vi "9239_1.vi"() -> ()   [LabVIEW 2014]
uses:
  <vilib>/Platform/TimedLoop/XDataNode/timing_clust.ctl
  <vilib>/Platform/TimedLoop/XDataNode/nitl_modes.ctl
  <vilib>/Platform/TimedLoop/XDataNode/wakeup.ctl
  <vilib>/Platform/TimedLoop/XDataNode/XDataNode.xnode
  <vilib>/Platform/TimedLoop/XDataNode/XDNodeRunTimeDep.lvlib
panel:
  out "已采样数量":dbl
  out "a1通道零漂采集":dynamicdata(graph)
  out "数据记录频率":dbl
  in  "路径":path
  in  "采样数":dbl=2000.0
  in  "采样率":dbl=2000.0
  out "波形图":dynamicdata(graph)
  out "时间":string
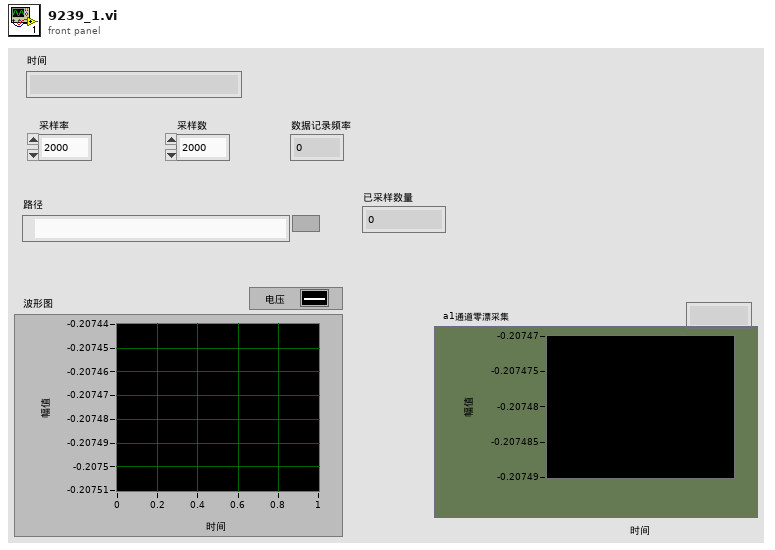
[diagram p1: front panel]
types:
  T1 = enum16{"open", "open or create", "create or replace", "create", "open (read-only)"}
  T2 = typedef "XDNodeRunTimeDep.lvlib/timing_clust.ctl" = cluster{"Expected End [f-1]":u64, "Actual End [f-1]":u64, "Finished Late? [f-1]":bool, "Expected End [i-1]":u64, "Actual End [i-1]":u64, "Finished Late? [i-1]":bool, "Expected Start [i]":u64, "Actual Start [i]":u64, "Expected Start [f]":u64, "Actual Start [f]":u64, "Source Name":string, "Structure Name":string, "Period":i64, "Deadline":i64, "Offset":i64, "Start":i64, "Priority":i32, "Timeout":i32, "Mode":T3, "Wakeup Reason":T4, "Error":errorcluster, "Source Type":string, "Secondary Source Type":string, "Global End Time":u64, "Global Start Time":u64, "Frame Duration":u64, "Iteration Duration":u64, "Assigned CPU":i32, "I/O Scan Engine Mode":u32}
  T3 = typedef "XDNodeRunTimeDep.lvlib/nitl_modes.ctl" = enum32{"No Change", "Process missed periods, maintain original phase", "Discard missed periods, maintain original phase", "Process missed periods, ignore original phase", "Discard missed periods, ignore original phase"}
  T4 = typedef "XDNodeRunTimeDep.lvlib/wakeup.ctl" = enum32{"Normal", "Aborted", "Asynchronous wakeup", "Timing source error", "Timed loop error", "Timeout"}
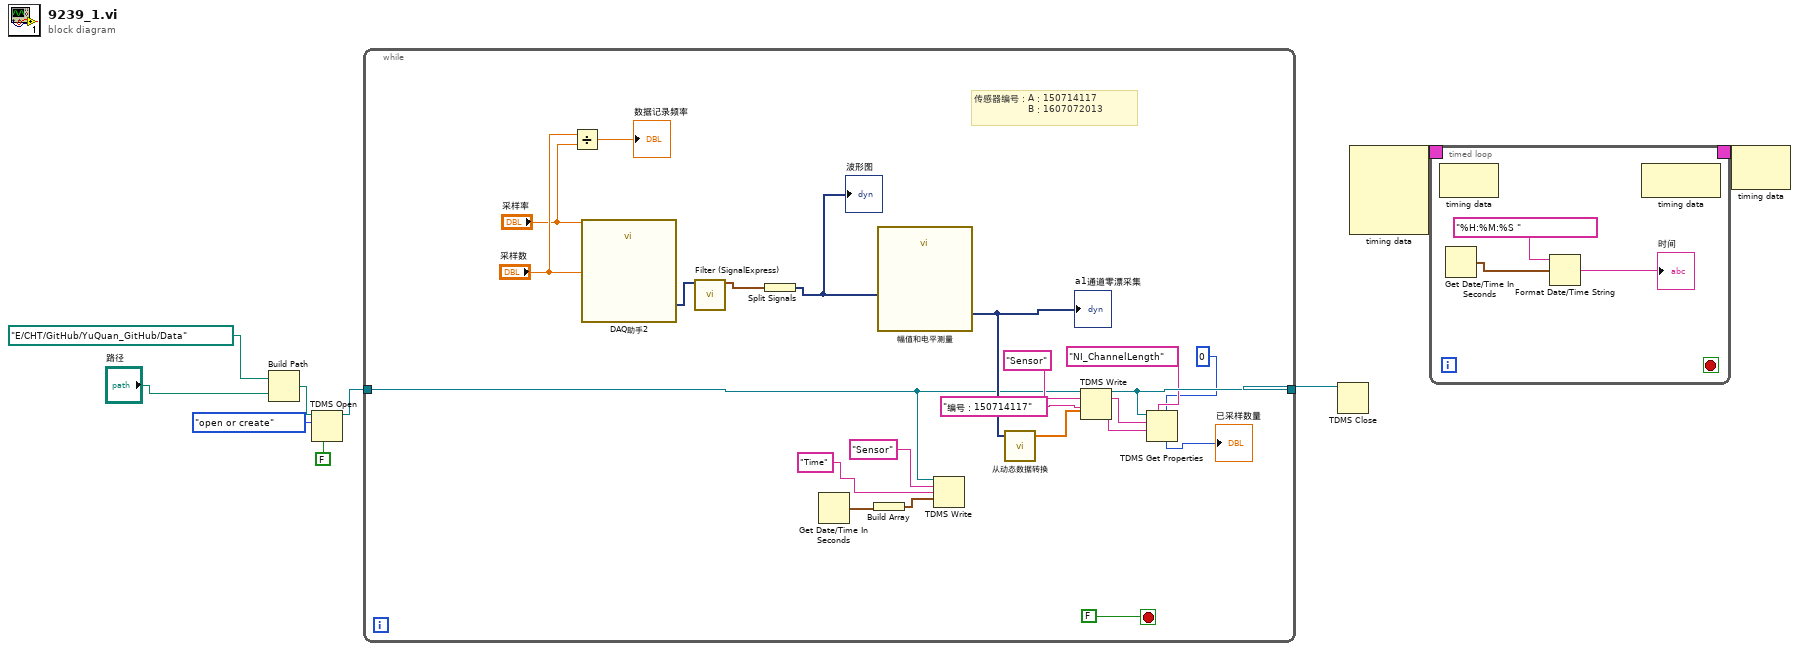
[diagram p0: block diagram]
diagram:
  n1 = Build Path(base path=path "E:/CHT/GitHub/YuQuan_GitHub/Data", name or relative path="路径") -> (appended path=w6:path)
  n2 = TDMS Open(6:FALSE ("disable buffering (T)"), 10:T1."open or create" ("operation"), 11:w6) -> (3:w4:refnum<k34>)  [unwired: 4 in, 1 out]
  n3 = while {
    tunnel: w4 -> [w12]
    tunnel: [w19] -> w3
    stop <- FALSE stop-if-true
    # "传感器编号：A：150714117\n                  B：1607072013"
    n4 = Divide(x="采样数", y="采样率") -> (x/y=→"数据记录频率":dbl)
    n5 = call "DAQ助手2"("速率"="采样率", "采样数"="采样数") -> ("data"=w27:dynamicdata)  [unwired: 14 in, 3 out]
    n6 = call "Filter (SignalExpress)"("input signals"=w27) -> ("filtered data"=w26:waveform(dbl)[])  [unwired: 17 in, 1 out]
    n7 = Split Signals(w26) -> (w25:dynamicdata)  [unwired: 1 in]
    "波形图" <- w25
    n8 = Get Date/Time In Seconds() -> (seconds since 1Jan1904=w14:timestamp)
    n9 = Build Array(w14) -> (w13:timestamp[])
    n10 = call "幅值和电平测量"("Signals"=w25) -> ("Mean (DC)"=w22:dynamicdata)  [unwired: 13 in, 1 out]
    "a1通道零漂采集" <- w22
    n11 = TDMS Write(0:w12, 5:"Sensor", 7:"Time", 9:w13) -> ()  [unwired: 2 in, 4 out]
    n12 = call "从动态数据转换"("Dynamic Data Type"=w22) -> ("Array"=w21:dbl[])  [unwired: 3 in]
    n13 = TDMS Write(0:w12, 5:"Sensor", 7:"编号：150714117", 9:w21) -> (4:w19:refnum<k34>, 6:w20:string, 8:w18:string)  [unwired: 2 in, 1 out]
    n14 = TDMS Get Properties(5:0, 7:"NI_ChannelLength", 9:w18, 10:w20, 11:w19) -> (4:→"已采样数量":i32)  [unwired: 1 in, 5 out]
  }
  n15 = TDMS Close(11:w3) -> ()  [unwired: 1 in, 2 out]
  n16 = node-c288() -> (w9:T2)  [unwired: 4 in]
  n17 = timed-loop {
    timing: w9 -> [_]
    timing-out: [_] -> w8
    stop <- _ stop-if-true
    n18 = node-c288() -> ()  [unwired: 1 in, 1 out]
    n19 = Get Date/Time In Seconds() -> (seconds since 1Jan1904=w34:timestamp)
    n20 = Format Date/Time String(time format string (%c)="%H:%M:%S ", seconds (now)=w34) -> (date/time string=→"时间":string)  [unwired: 1 in]
    n21 = node-c288() -> ()  [unwired: 1 in, 1 out]
  }
  n22 = node-c288(w8) -> ()  [unwired: 1 out]
